vi "F2Csub.vi"(1 "Numeric 2":dbl, 2 "Temperature (F)":dbl) -> (0 "Numeric":dbl)   [LabVIEW 2013]
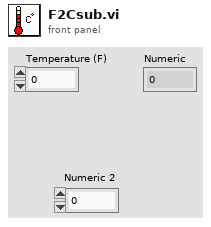
[diagram p1: front panel]
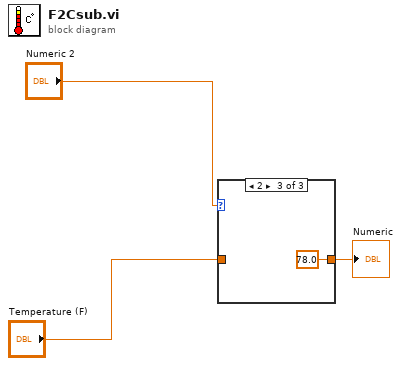
[diagram p0: block diagram]
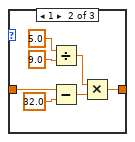
[diagram p3: hidden frame]
diagram:
  n1 = case shown="2" "Numeric 2" {
    tunnel: [w4 w9 78.0 ("Temperature (F)")] -> w3
    tunnel: "Temperature (F)" -> [w4 w5 _]
    frame 0, Default {
    }
    frame 1 {
      n2 = Divide(x=5.0, y=9.0) -> (x/y=w11:dbl)
      n3 = Subtract(x=w5, y=32.0) -> (x-y=w10:dbl)
      n4 = Multiply(x=w11, y=w10) -> (x*y=w9:dbl)
    }
    frame 2 {
    }
  }
  "Numeric" <- w3
